vi "FGV_camera_status.vi"(6 "Enum":enum16{"Init", "Read", "Write"}(ring), 10 "Write":T1) -> (2 "Read":T1)   [LabVIEW 2024, in "Keyence_VS150.lvlib"]
uses:
  Keyence_VS150.lvlib
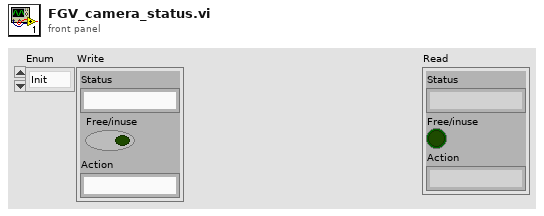
[diagram p1: front panel]
types:
  T1 = cluster{"Status":string, "Free/inuse":bool, "Action":string}
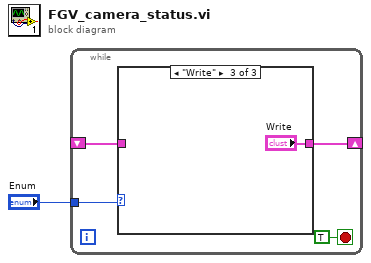
[diagram p0: block diagram]
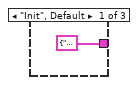
[diagram p2: hidden frame]
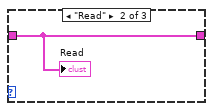
[diagram p3: hidden frame]
diagram:
  n1 = while {
    tunnel: "Enum" -> [w4]
    shift-right: [w3] -> _
    shift-left: _ -> [w2]
    stop <- TRUE stop-if-true
    n2 = case shown="\"Write\"" w4 {
      tunnel: [T1 {"Status"="", "Free/inuse"=FALSE, "Action"=""} w7 "Write"] -> w3
      tunnel: w2 -> [_ w7 _]
      frame "Init", Default {
      }
      frame "Read" {
        "Read" <- w7
      }
      frame "Write" {
      }
    }
  }
